vi "Register User Events.vi"(8 "error in (no error)":errorcluster, 11 "SongBrowserActor in":refnum<class "SongBrowserActor.lvclass">) -> (0 "error out":errorcluster, 3 "SongBrowserActor out":refnum<class "SongBrowserActor.lvclass">, 5 "Event Registration Refnum":refnum<event-registration>, 7 "Exit Event":refnum<user-event>)   [LabVIEW 2015, in "SongBrowserActor.lvlib" / "SongBrowserActor.lvclass"]
uses:
  SongBrowserActor.lvclass
  builds/xctls/Artist Browser/Artist Browser.lvlibp/app/controls/Music Library Element Display.ctl
  builds/xctls/Artist Browser/Artist Browser.lvlibp/file/MusicElement/Song/Song Duration.ctl
  builds/xctls/Song Browser/Song Browser.lvlibp/app/controls/Queue Song Display.ctl
  builds/xctls/Song Browser/Song Browser.lvlibp/file/MusicElement/Song/Song Duration.ctl
  builds/xctls/Song Browser/Song Browser.lvlibp/app/controls/Dequeue Control.ctl
  SongBrowserActor.lvclass/SongBrowserActor.ctl
  builds/xctls/Artist Browser/Artist Browser.lvlibp/app/xctls/Artist Browser/Artist Browser.xctl
  builds/xctls/Song Browser/Song Browser.lvlibp/app/xctls/Song Browser/Song Browser.xctl
  builds/xctls/Album Browser/Album Browser.lvlibp/app/xctls/Album Browser/Album Browser/Album Browser.xctl
  builds/xctls/Song Browser/Song Browser.lvlibp
  builds/xctls/Song Browser/Song Browser.lvlibp/file/MusicElement/Song/Song.lvclass
  builds/xctls/Artist Browser/Artist Browser.lvlibp/file/MusicElement/Song/Song.lvclass
  builds/xctls/Artist Browser/Artist Browser.lvlibp
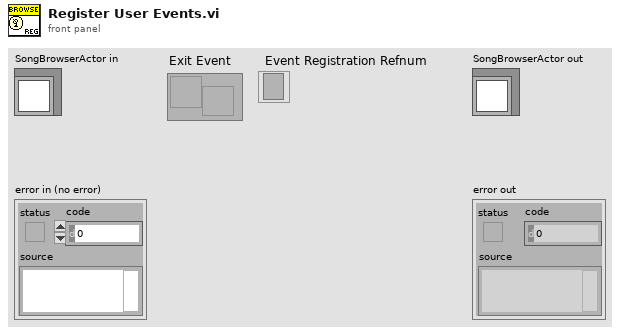
[diagram p1: front panel]
types:
  T1 = typedef "Artist Browser.lvlibp/Music Library Element Display.ctl" = cluster{"Name":string, "Details":string, "Duration (s)":T2, "Click":bool}
  T2 = typedef "Artist Browser.lvlibp/Song.lvclass/Song Duration.ctl" = timestamp
  T3 = typedef "Song Browser.lvlibp/Queue Song Display.ctl" = cluster{"Song Name":string, "Artist":string, "Album":string, "Duration (s)":T4, "UID":string, "Dequeue":T5}
  T4 = typedef "Song Browser.lvlibp/Song.lvclass/Song Duration.ctl" = timestamp
  T5 = typedef "Song Browser.lvlibp/Dequeue Control.ctl" = bool
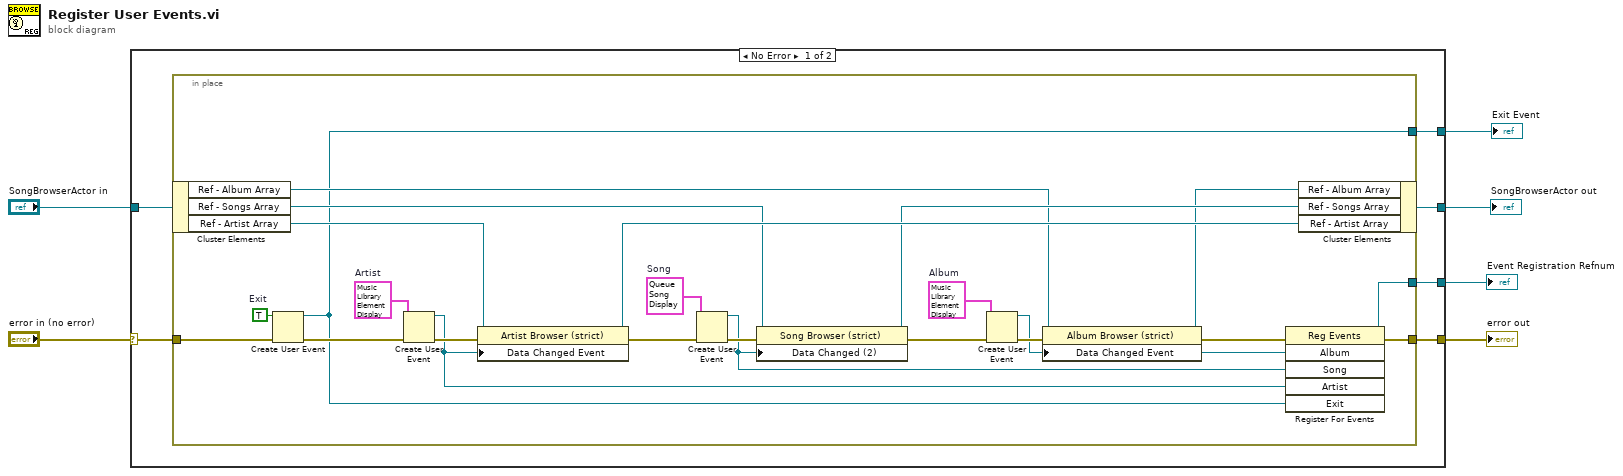
[diagram p0: block diagram]
diagram:
  n1 = case shown="No Error" "error in (no error)" {
    selector: "error in (no error)" -> [w12 w38]
    tunnel: [w11 w38] -> w5
    tunnel: [w9 w37] -> w3
    tunnel: "SongBrowserActor in" -> [w10 w37]
    tunnel: [w8 _] -> w2
    tunnel: [w7 _] -> w1
    frame No Error {
      n2 = in-place {
        in-place-border: w12 -> [w16]
        in-place-border: [w18] -> w11
        in-place-border: [w14] -> w8
        in-place-border: [w13] -> w7
        w17 = TRUE  # Exit
        w24 = T1 {"Name"="", "Details"="", "Duration (s)"=timestamp(0 s since 1904-01-01), "Click"=FALSE}  # Album
        w32 = T1 {"Name"="", "Details"="", "Duration (s)"=timestamp(0 s since 1904-01-01), "Click"=FALSE}  # Artist
        w33 = T3 {"Song Name"="", "Artist"="", "Album"="", "Duration (s)"=timestamp(0 s since 1904-01-01), "UID"="", "Dequeue"=FALSE}  # Song
        n3 = in-place-cluster #1(w10) -> ("Ref - Album Array"=w23:refnum<vi>, "Ref - Songs Array"=w29:refnum<vi>, "Ref - Artist Array"=w31:refnum<vi>)
        n4 = Create User Event(user event datatype=w17, error in=w16) -> (user event=w13:refnum<user-event>, error out=w15:errorcluster)
        n5 = Create User Event(user event datatype=w32, error in=w15) -> (user event=w19:refnum<user-event>, error out=w36:errorcluster)
        n6 = property on="Property Node" class="Artist Browser (strict)"(reference=w31, error in=w36, "Data Changed Event"=w19) -> (reference out=w30:refnum<vi>, error out=w34:errorcluster)
        n7 = Create User Event(user event datatype=w33, error in=w34) -> (user event=w20:refnum<user-event>, error out=w35:errorcluster)
        n8 = property on="Property Node" class="Song Browser (strict)"(reference=w29, error in=w35, "Data Changed (2)"=w20) -> (reference out=w28:refnum<vi>, error out=w26:errorcluster)
        n9 = Create User Event(user event datatype=w24, error in=w26) -> (user event=w21:refnum<user-event>, error out=w27:errorcluster)
        n10 = property on="Property Node" class="Album Browser (strict)"(reference=w23, error in=w27, "Data Changed Event"=w21) -> (reference out=w25:refnum<vi>, error out=w22:errorcluster)
        n11 = register-events(error in=w22, w21, w20, w19, w13) -> (reference out=w14:refnum<event-registration>, error out=w18:errorcluster)  [unwired: 1 in]
        n12 = in-place-cluster #1("Ref - Album Array"=w25, "Ref - Songs Array"=w28, "Ref - Artist Array"=w30) -> (w9:refnum<class "SongBrowserActor.lvclass">)
      }
    }
    frame Error {
    }
  }
  "error out" <- w5
  "SongBrowserActor out" <- w3
  "Event Registration Refnum" <- w2
  "Exit Event" <- w1
